vi "File_AddPathsToArrayWithoutDuplicates.vi"(1 "Paths in":path[](array[path]), 4 "Paths to be added":path[](array[path])) -> (15 "Paths out":path[](array[path]), 18 "Added paths":path[](array[path]))   [LabVIEW 2020]
doc: "Adds paths to array, but will not duplicate any path."
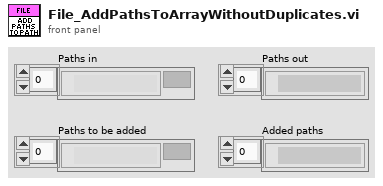
[diagram p1: front panel]
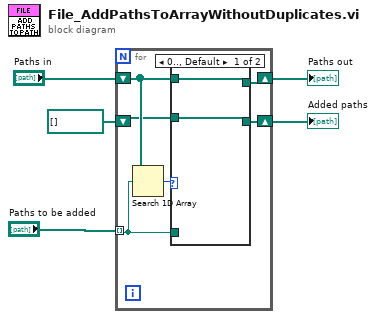
[diagram p0: block diagram]
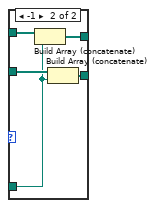
[diagram p2: hidden frame]
diagram:
  n1 = for {
    shift-right: [w9] -> w4
    shift-left: "Paths in" -> [w10]
    tunnel: "Paths to be added" -> [w8] mode=indexing
    shift-right: [w6] -> w1
    shift-left: path[] [] ("Paths in") -> [w7]
    n2 = Search 1D Array(1D array=w10, element=w8) -> (index of element=w11:i32)  [unwired: 1 out]
    n3 = case shown="0.., Default" w11 {
      tunnel: w10 -> [w13 w18]
      tunnel: [w13 w17] -> w9
      tunnel: w8 -> [_ w14]
      tunnel: w7 -> [w12 w16]
      tunnel: [w12 w15] -> w6
      frame 0.., Default {
      }
      frame -1 {
        n4 = Build Array (concatenate)(w18, w14) -> (w17:path[])
        n5 = Build Array (concatenate)(w16, w14) -> (w15:path[])
      }
    }
  }
  "Paths out" <- w4
  "Added paths" <- w1
